vi "Current slew rate with scope.vi"() -> ()   [LabVIEW 2021]
uses:
  <instrlib>/niDCPower/nidcpower.llb/niDCPower Wait For Event - Event.ctl
  <instrlib>/niDCPower/nidcpower.llb/niDCPower Source Mode.ctl
  <instrlib>/niDCPower/nidcpower.llb/niDCPower Output Function.ctl
  <instrlib>/niDCPower/nidcpower.llb/niDCPower Aperture Time Units.ctl
  <instrlib>/niScope/Controls/niScope trigger slope.ctl
  <instrlib>/niScope/Utility/niScope Get Channel Name From String.vi
  <instrlib>/niScope/Configure/Trigger/niScope Configure Trigger Digital.vi
  <instrlib>/niDCPower/nidcpower.llb/niDCPower Configure Digital Edge Measure Trigger With Channels.vi
  <instrlib>/niScope/Acquire/Fetch/niScope Fetch WDT.vi
panel:
  in  "MeasGraphs":T1(tab)
  out "CurrentV/STime":waveform(dbl)(graph) caption="Load Transient"
  in  "SourceOutput Voltage v/s Time":string="SOURCE VOLTAGE vs TIME"
  out "ScopeAmplitudeV/STime":waveform(dbl)(graph) caption="Load Transient"
  in  "ScopeOutput Voltage v/s Time":string="SCOPE AMPLITUDE vs TIME"
  in  "error in":errorcluster caption="error in (no error)"
  out "error out":errorcluster
  in  "Source transient response":i32(ring)=1041 items=["Slow"=1041, "Normal"=1038, "Fast"=1039, "Custom"=1042]
  in  "MeasConfigurations":enum32{"Source Config", "Scope Config"}(tab)
  in  "TransientResponseTab":T2(tab)
  in  "Transient response":enum16{"Slow", "Normal", "Fast", "Custom"}(ring)=enum."Fast" caption="TRANSIENT RESPONSE"
  in  "Source current gain bandwidth":dbl=2000.0 caption="GAIN BANDWIDTH" format="%#_6pHz"
  in  "Source current compensation frequency":dbl=3530.0 caption="COMP. FREQUENCY" format="%#_6pHz"
  in  "Source current pole-zero ratio":dbl=2.0 caption="POLE-ZERO RATIO"
  in  "Source update rate":dbl=100000.0 caption="UPDATE RATE" format="%#_6pS/s"
  in  "Source sense":i32(ring)=1009 caption="SENSE" items=["Local"=1008, "Remote"=1009]
  in  "Source current C2 time":dbl=0.005 caption="TIME for C2" format="%#_6ps"
  in  "Source current C1 time":dbl=0.005 caption="TIME for C1" format="%#_6ps"
  in  "Source current slew rate":dbl=500.0 caption="CURRENT SLEW RATE" format="%#_6pA/s"
  in  "Source voltage limit range":dbl=20.0 caption="VOLTAGE LIMIT RANGE" format="%#_6pV"
  in  "Source current level range":dbl=3.0 caption="CURRENT LEVEL RANGE" format="%#_6pA"
  in  "Source current set point 2(C2)":dbl=3.0 caption="CURRENT SET POINT 2" format="%#_6pA"
  in  "Source current set point 1(C1)":dbl caption="CURRENT SET POINT 1" format="%#_6pA"
  in  "Source resource name":refnum<k15> caption="RESOURCE NAME"
  in  "Source SourceAdapt":string="Voltage SourceAdapt Parameters"
  in  "Source sample rate":dbl=1800000.0 caption="SAMPLE RATE" format="%#_6pS/s"
  in  "Scope enable/disable":bool caption="Scope Enable/Disable"
  in  "Scope vertical range":dbl=10.0 caption="VERTICAL RANGE"
  in  "Scope resourceName":refnum<k15> caption="RESOURCE NAME"
  in  "Scope probe attenuation":dbl=1.0 caption="PROBE ATTENUATION"
  in  "Scope sample rate":dbl=1800000.0 caption="SAMPLE RATE" format="%#_6pHz"
  in  "Scope output channel name":string="0" caption="INPUT CHANNEL NAME"
  in  "Scope vertical coupling":enum32{"AC", "DC"}(ring)=enum."DC" caption="VERTICAL COUPLING"
  # "CURRENT SLEW RATE"
  # "-"
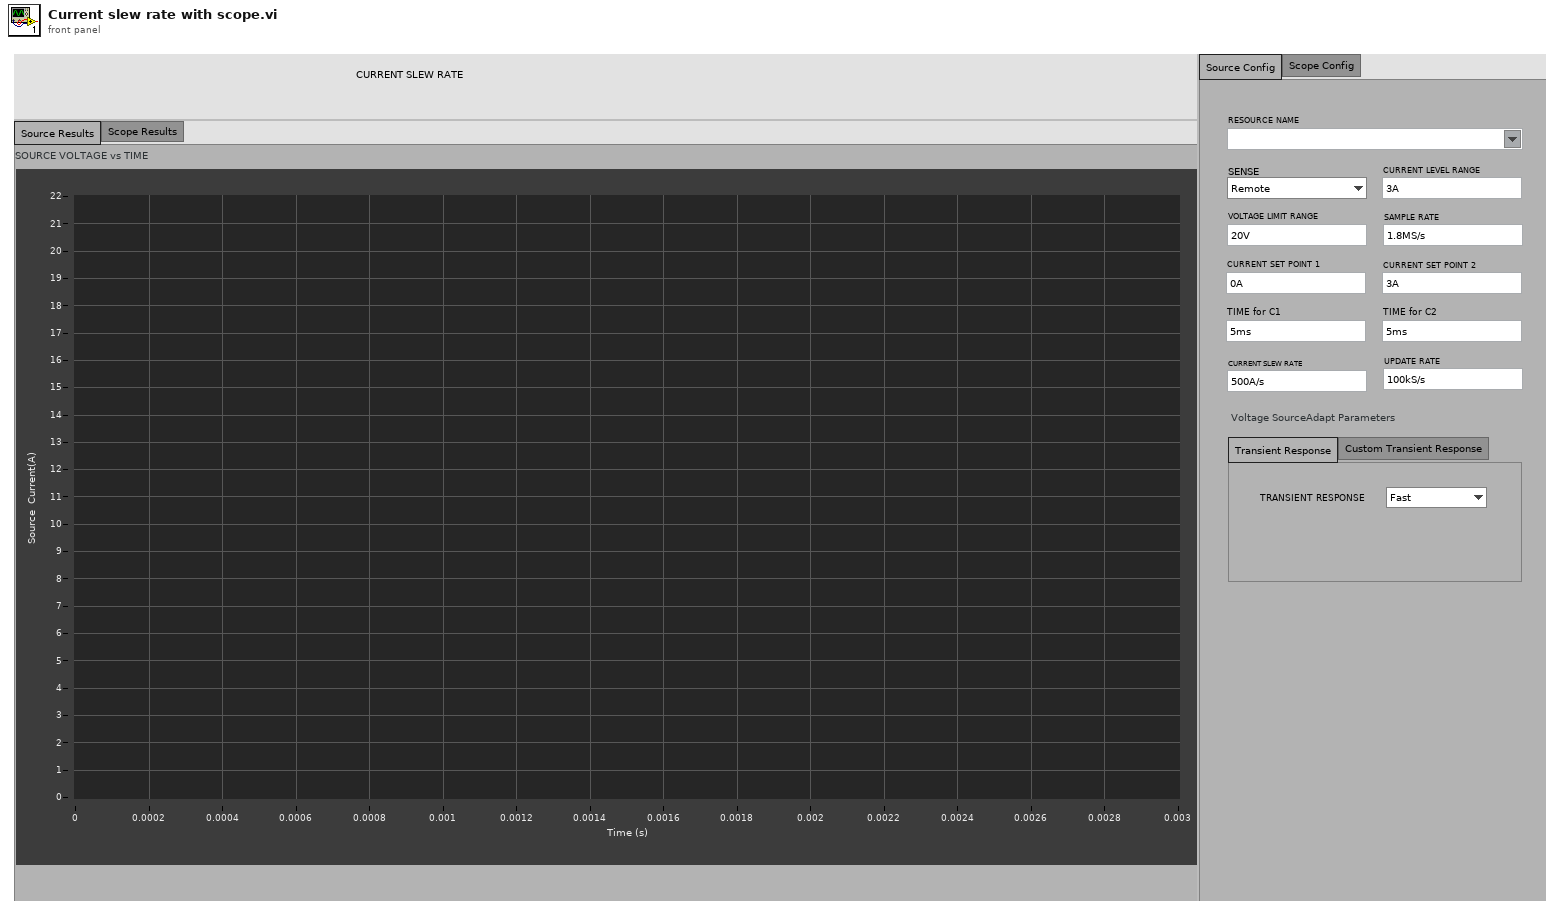
[diagram p1: front panel]
types:
  T1 = enum32{"Source Results", "Scope Results", "Hidden Controls"}
  T2 = enum32{"Transient Response", "Custom Transient Response"}
  T3 = typedef "niDCPower Aperture Time Units.ctl" = i32
  T4 = typedef "niDCPower Output Function.ctl" = i32
  T5 = typedef "niDCPower Wait For Event - Event.ctl" = i32
  T6 = typedef "niDCPower Source Mode.ctl" = i32
  T7 = typedef "niScope trigger slope.ctl" = i32
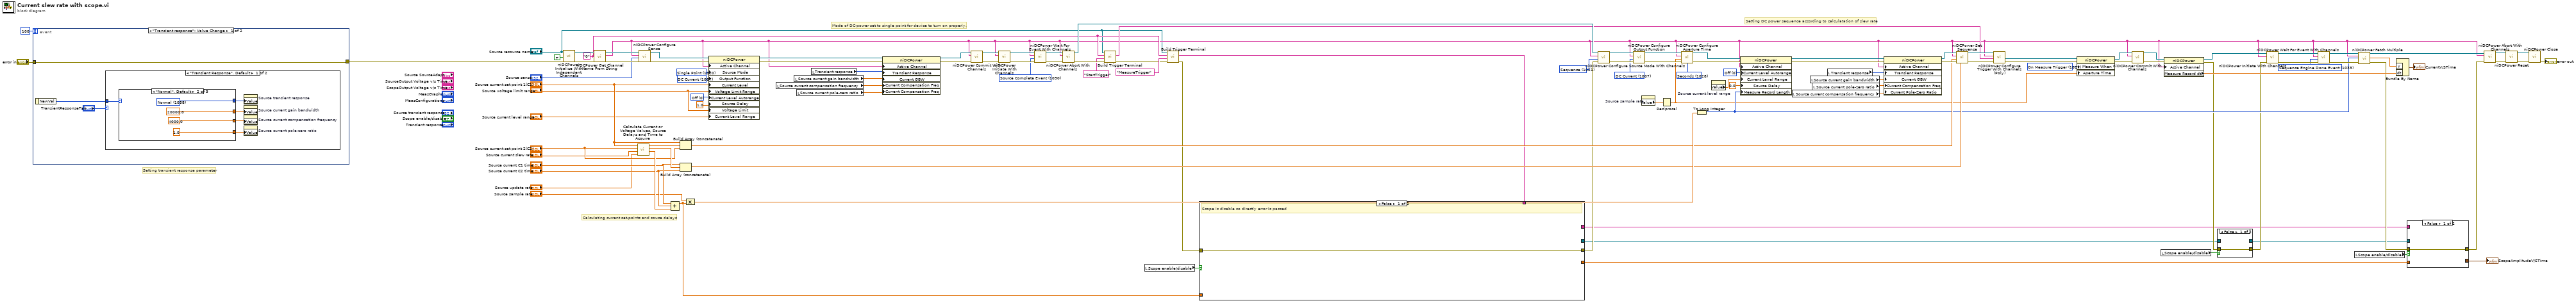
[diagram p0: block diagram]
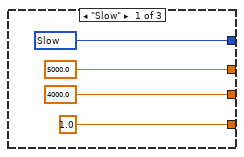
[diagram p2: hidden frame]
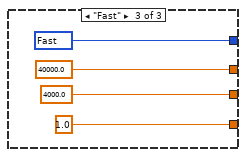
[diagram p3: hidden frame]
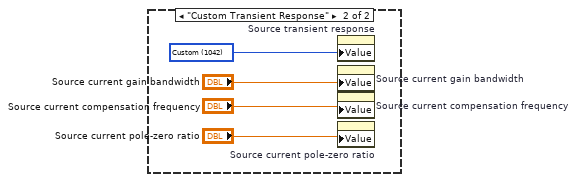
[diagram p4: hidden frame]
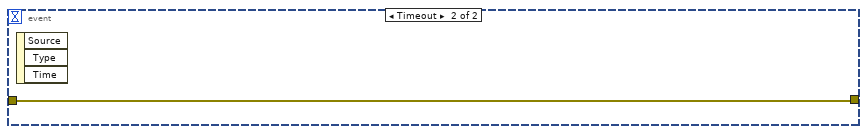
[diagram p5: hidden frame]
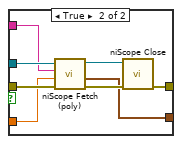
[diagram p6: hidden frame]
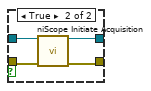
[diagram p7: hidden frame]
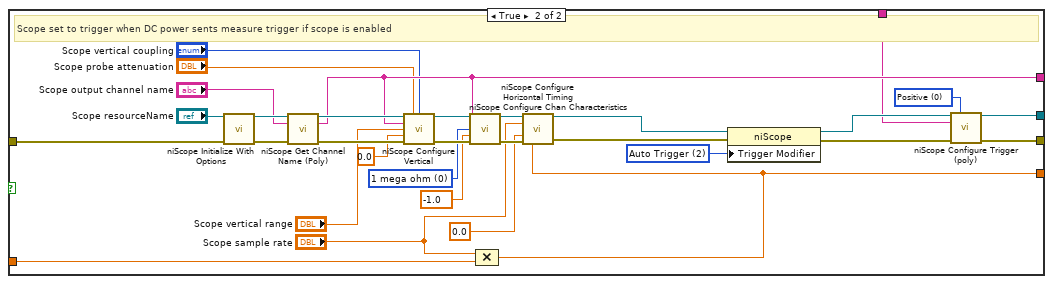
[diagram p8: hidden frame]
diagram:
  w73 = 1027 items=["Automatically after Source Complete"=1025, "On Demand"=1026, "On Measure Trigger"=1027] ("Measurement:Advanced:Measure When")
  w76 = 0 items=["Off", "On"] ("Source:DC Current:Current Level Autorange")
  w81 = T3 1028 items=["Seconds"=1028, "Powerline Cycles"=1029] ("aperture time units")
  w80 = T4 1007 items=["DC Voltage"=1006, "DC Current"=1007, "Pulse Voltage"=1049, "Pulse Current"=1050] ("output function")
  w82 = T5 1033 items=["Source Complete Event"=1030, "Measure Complete Event"=1031, "Sequence Iteration Complete Event"=1032, "Sequence Engine Done Event"=1033, "Pulse Complete Event"=1051, "Ready For Pulse Trigger Event"=1052] ("event")
  w83 = T6 1021 items=["Single Point"=1020, "Sequence"=1021] ("source mode")
  w44 = "0" ("index")
  w104 = 0 items=["Off", "On"] ("Source:DC Current:Current Level Autorange")
  w113 = T5 1030 items=["Source Complete Event"=1030, "Measure Complete Event"=1031, "Sequence Iteration Complete Event"=1032, "Sequence Engine Done Event"=1033, "Pulse Complete Event"=1051, "Ready For Pulse Trigger Event"=1052] ("event")
  w116 = 1007 items=["DC Voltage"=1006, "DC Current"=1007, "Pulse Voltage"=1049, "Pulse Current"=1050] ("Source:Output Function")
  w117 = 1020 items=["Single Point"=1020, "Sequence"=1021] ("Source:Source Mode")
  # "Calculating current set-points and souce delays"
  # "Setting DC power sequence according to calculatation of slew rate"
  # "Mode of DC-power set to single point for device to turn on properly."
  # "Setting transient response parameter"
  n1 = event shown="[0] \"Transient response\": Value Change" {
    selector: _ -> [_ _]
    dyn-events: _ -> [_ _]
    timeout: 100 -> [_ _]
    tunnel: [w120 w142] -> w1
    tunnel: "error in" -> [w120 w142]
    event "Transient response": Value Change {
      n2 = event-data() -> ("NewVal"=w119:enum16{"Slow", "Normal", "Fast", "Custom"})  [unwired: 1 in]
      n3 = case shown="\"Transient Response\", Default" "TransientResponseTab" {
        tunnel: w119 -> [w121 _]
        frame "Transient Response", Default {
          n4 = case shown="\"Normal\", Default" w121 {
            tunnel: [w129 w133 w137] -> w125
            tunnel: [5000.0 ("Source voltage gain bandwidth") 20000.0 ("Source voltage gain bandwidth") 40000.0 ("Source voltage gain bandwidth")] -> w124
            tunnel: [4000.0 ("Source voltage compensation frequency") 4000.0 ("Source voltage compensation frequency") 4000.0 ("Source voltage compensation frequency")] -> w122
            tunnel: [1.0 ("Source voltage pole-zero ratio") 1.0 ("Source voltage pole-zero ratio") 1.0 ("Source voltage pole-zero ratio")] -> w123
            frame "Slow" {
              w129 = 1041 items=["Slow"=1041, "Normal"=1038, "Fast"=1039, "Custom"=1042] ("Source transient response")
            }
            frame "Normal", Default {
              w133 = 1038 items=["Slow"=1041, "Normal"=1038, "Fast"=1039, "Custom"=1042] ("Source transient response")
            }
            frame "Fast" {
              w137 = 1039 items=["Slow"=1041, "Normal"=1038, "Fast"=1039, "Custom"=1042] ("Source transient response")
            }
          }
          n5 = property on="Source transient response" class="Ring (strict)"("Value"=w125) -> ()  [unwired: 2 in, 2 out]
          n6 = property on="Source current gain bandwidth" class="DigNum (strict)"("Value"=w124) -> ()  [unwired: 2 in, 2 out]
          n7 = property on="Source current compensation frequency" class="DigNum (strict)"("Value"=w122) -> ()  [unwired: 2 in, 2 out]
          n8 = property on="Source current pole-zero ratio" class="DigNum (strict)"("Value"=w123) -> ()  [unwired: 2 in, 2 out]
        }
        frame "Custom Transient Response" {
          w141 = 1042 items=["Slow"=1041, "Normal"=1038, "Fast"=1039, "Custom"=1042] ("Source transient response")
          n9 = property on="Source transient response" class="Ring (strict)"("Value"=w141) -> ()  [unwired: 2 in, 2 out]
          n10 = property on="Source current gain bandwidth" class="DigNum (strict)"("Value"="Source current gain bandwidth") -> ()  [unwired: 2 in, 2 out]
          n11 = property on="Source current compensation frequency" class="DigNum (strict)"("Value"="Source current compensation frequency") -> ()  [unwired: 2 in, 2 out]
          n12 = property on="Source current pole-zero ratio" class="DigNum (strict)"("Value"="Source current pole-zero ratio") -> ()  [unwired: 2 in, 2 out]
        }
      }
    }
    event Timeout {
      n13 = event-data() -> ()  [unwired: 1 in, 3 out]
    }
  }
  n14 = call <instrlib>:"niDCPower Initialize With Independent Channels.vi"("error in (no error)"=w1, "reset (false)"=TRUE, "resource name"="Source resource name") -> ("error out"=w98:errorcluster, "instrument handle out"=w101:refnum<k15>)  [unwired: 7 in]
  n15 = call <instrlib>:"niDCPower Get Channel Name From String.vi"("error in (no error)"=w98, "index"=w44, "instrument handle"=w101) -> ("error out"=w99:errorcluster, "name"=w37:string, "instrument handle out"=w100:refnum<k15>)  [unwired: 6 in]
  n16 = call "Calculate Current or Voltage Values, Source Delays and Time to Acquire.vi"("Update Rate (S/sec)"="Source update rate", "Current/voltage slew rate (AorV/sec)"="Source current slew rate", "Current/voltage end point (A/V)"="Source current set point 2(C2)", "Current/voltage start point  (A/V)"="Source current set point 1(C1)") -> ("Time to acquire (sec)"=w36:dbl, "Source delays (sec)"=w35:dbl[], "Current/voltage values"=w34:dbl[])  [unwired: 5 in]
  n17 = call <instrlib>:"niDCPower Configure Sense.vi"("error in (no error)"=w99, "sense"="Source sense", "channel name"=w37, "instrument handle"=w100) -> ("error out"=w109:errorcluster, "instrument handle out"=w110:refnum<k15>)  [unwired: 6 in]
  n18 = Compound Arithmetic op=ADD("Source current C1 time", "Source current C2 time", w36) -> (w47:dbl)
  n19 = Build Array (concatenate)("Source current set point 1(C1)", w34, "Source current set point 2(C2)") -> (w66:dbl[])
  n20 = Build Array (concatenate)("Source current C1 time", w35, "Source current C2 time") -> (w67:dbl[])
  n21 = Compound Arithmetic op=MULTIPLY("Source sample rate", w47) -> (w90:dbl)
  n22 = property class="niDCPower"(reference=w110, error in=w109, "Active Channel"=w37, "Source Mode"=w117, "Output Function"=w116, "Current Level"="Source current set point 1(C1)", "Voltage Limit Range"="Source voltage limit range", "Current Level Autorange"=w104, "Source Delay"=1.0 ("Source:Advanced:Source Delay"), "Voltage Limit"="Source voltage limit range", "Current Level Range"="Source current level range") -> (reference out=w106:refnum<k15>, error out=w105:errorcluster)
  n23 = local read "Source current compensation frequency"() -> (w12:dbl)
  n24 = local read "Source current gain bandwidth"() -> (w13:dbl)
  n25 = local read "Source current pole-zero ratio"() -> (w11:dbl)
  n26 = local read "Transient response"() -> (w10:enum16{"Slow", "Normal", "Fast", "Custom"})
  n27 = property class="niDCPower"(reference=w106, error in=w105, "Active Channel"=w37, "Transient Response"=w10, "Current GBW"=w13, "Current Compensation Freq"=w12, "Current Compensation Freq"=w11) -> (reference out=w103:refnum<k15>, error out=w102:errorcluster)
  n28 = call <instrlib>:"niDCPower Commit With Channels.vi"("error in (no error)"=w102, "channel name"=w37, "instrument handle"=w103) -> ("error out"=w107:errorcluster, "instrument handle out"=w108:refnum<k15>)  [unwired: 7 in]
  n29 = call <instrlib>:"niDCPower Initiate With Channels.vi"("error in (no error)"=w107, "channel name"=w37, "instrument handle"=w108) -> ("error out"=w115:errorcluster, "instrument handle out"=w114:refnum<k15>)  [unwired: 7 in]
  n30 = call <instrlib>:"niDCPower Wait For Event With Channels.vi"("error in (no error)"=w115, "event"=w113, "channel name"=w37, "instrument handle"=w114) -> ("error out"=w112:errorcluster, "instrument handle out"=w111:refnum<k15>)  [unwired: 6 in]
  n31 = call <instrlib>:"niDCPower Abort With Channels.vi"("error in (no error)"=w112, "channel name"=w37, "instrument handle"=w111) -> ("error out"=w58:errorcluster, "instrument handle out"=w68:refnum<k15>)  [unwired: 7 in]
  n32 = call "Build Trigger Terminal.vi"("error in (no error)"=w58, "Trigger/Event Name"="StartTrigger" ("Trigger Type"), "Channel Name"=w44, "Resource Name"="Source resource name") -> ("error out"=w30:errorcluster, "Terminal Name"=w57:string)  [unwired: 6 in]
  n33 = local read "Scope enable/disable"() -> (w15:bool)
  n34 = call "Build Trigger Terminal.vi"("error in (no error)"=w30, "Trigger/Event Name"="MeasureTrigger", "Channel Name"=w44, "Resource Name"="Source resource name") -> ("error out"=w45:errorcluster, "Terminal Name"=w33:string)  [unwired: 6 in]
  n35 = case shown="False" w15 {
    tunnel: [w143 w156] -> w55
    tunnel: [_ w155] -> w50
    tunnel: [_ w154] -> w48
    tunnel: w47 -> [_ w153]
    tunnel: [_ w152] -> w46
    tunnel: w45 -> [w143 w151]
    tunnel: w33 -> [_ w150]
    frame False {
      # "Scope is disable so directly error is passed"
    }
    frame True {
      w163 = 2 items=["None"=1, "Auto Trigger"=2] ("Trigger Modifier")
      w159 = u32 0 items=["1 mega ohm"=0, "50 ohms"=2] ("Input Impedance")
      w160 = T7 0 items=["Positive", "Negative"] ("trigger slope")
      # "Scope set to trigger when DC power sents measure trigger if scope is enabled"
      n36 = call <instrlib>:"niScope Initialize With Options.vi"("resource name"="Scope resourceName", "error in"=w151) -> ("instrument handle"=w174:refnum<k15>, "error out"=w173:errorcluster)  [unwired: 12 in]
      n37 = call-poly <instrlib>:"niScope Get Channel Name (Poly).vi"("instrument handle"=w174, "index"="Scope output channel name", "error in"=w173) -> ("instrument handle out"=w162:refnum<k15>, "channel name"=w154:string, "error out"=w161:errorcluster)  [unwired: 10 in]
      n38 = call <instrlib>:"niScope Configure Vertical.vi"("instrument handle"=w162, "probe attenuation"="Scope probe attenuation", "vertical coupling"="Scope vertical coupling", "channels"=w154, "vertical range"="Scope vertical range", "vertical offset"=0.0, "error in"=w161) -> ("instrument handle out"=w172:refnum<k15>, "error out"=w171:errorcluster)  [unwired: 7 in]
      n39 = call <instrlib>:"niScope Configure Chan Characteristics.vi"("instrument handle"=w172, "channels"=w154, "input impedance"=w159, "maximum input frequency"=-1.0 ("Maximum Input Frequency"), "error in"=w171) -> ("instrument handle out"=w169:refnum<k15>, "error out"=w170:errorcluster)  [unwired: 9 in]
      n40 = Compound Arithmetic op=MULTIPLY("Scope sample rate", w153) -> (w152:dbl)
      n41 = call <instrlib>:"niScope Configure Horizontal Timing.vi"("instrument handle"=w169, "min sample rate"="Scope sample rate", "reference position"=0.0 ("Reference Position"), "error in"=w170, "min record length"=w152) -> ("instrument handle out"=w166:refnum<k15>, "error out"=w165:errorcluster)  [unwired: 9 in]
      n42 = property on="Property Node" class="niScope"(reference=w166, error in=w165, "Trigger Modifier"=w163) -> (reference out=w157:refnum<k15>, error out=w164:errorcluster)
      n43 = call-poly <instrlib>:"niScope Configure Trigger (poly).vi"("instrument handle"=w157, "trigger slope"=w160, "trigger source"=w150, "error in"=w164) -> ("instrument handle out"=w155:refnum<k15>, "error out"=w156:errorcluster)  [unwired: 10 in]
    }
  }
  n44 = call <instrlib>:"niDCPower Configure Source Mode With Channels.vi"("error in (no error)"=w55, "source mode"=w83, "channel name"=w37, "instrument handle"=w68) -> ("error out"=w86:errorcluster, "instrument handle out"=w85:refnum<k15>)  [unwired: 6 in]
  n45 = call <instrlib>:"niDCPower Configure Output Function.vi"("error in (no error)"=w86, "output function"=w80, "channel name"=w37, "instrument handle"=w85) -> ("error out"=w88:errorcluster, "instrument handle out"=w87:refnum<k15>)  [unwired: 6 in]
  n46 = property on="Source sample rate" class="DigNum (strict)"() -> ("Value"=w2:dbl)  [unwired: 2 in, 2 out]
  n47 = Reciprocal(x=w2) -> (1/x=w32:dbl)
  n48 = call <instrlib>:"niDCPower Configure Aperture Time.vi"("aperture time units"=w81, "error in (no error)"=w88, "aperture time"=w32, "channel name"=w37, "instrument handle"=w87) -> ("error out"=w78:errorcluster, "instrument handle out"=w77:refnum<k15>)  [unwired: 5 in]
  n49 = To Long Integer(number=w90) -> (32bit integer=w63:i32)
  n50 = property on="Source current level range" class="DigNum (strict)"() -> ("Value"=w3:dbl)  [unwired: 2 in, 2 out]
  n51 = property class="niDCPower"(reference=w77, error in=w78, "Active Channel"=w37, "Current Level Autorange"=w76, "Current Level Range"=w3, "Source Delay"=0.0 ("Source:Advanced:Source Delay"), "Measure Record Length"=w63) -> (reference out=w94:refnum<k15>, error out=w95:errorcluster)
  n52 = local read "Source current compensation frequency"() -> (w7:dbl)
  n53 = local read "Source current gain bandwidth"() -> (w9:dbl)
  n54 = local read "Source current pole-zero ratio"() -> (w8:dbl)
  n55 = local read "Transient response"() -> (w14:enum16{"Slow", "Normal", "Fast", "Custom"})
  n56 = property class="niDCPower"(reference=w94, error in=w95, "Active Channel"=w37, "Transient Response"=w14, "Current GBW"=w9, "Current Compensation Freq"=w8, "Current Pole-Zero Ratio"=w7) -> (reference out=w96:refnum<k15>, error out=w97:errorcluster)
  n57 = call <instrlib>:"niDCPower Set Sequence.vi"("source delays"=w67, "error in (no error)"=w97, "values"=w66, "channel name"=w37, "instrument handle"=w96) -> ("error out"=w74:errorcluster, "instrument handle out"=w75:refnum<k15>)  [unwired: 5 in]
  n58 = call-poly <instrlib>:"niDCPower Configure Trigger With Channels (Poly).vi"("error in (no error)"=w74, "input terminal"=w57, "channel name"=w37, "instrument handle"=w75) -> ("error out"=w70:errorcluster, "instrument handle out"=w72:refnum<k15>)  [unwired: 6 in]
  n59 = property class="niDCPower"(reference=w72, error in=w70, "Measure When"=w73, "Aperture Time"=w32) -> (reference out=w71:refnum<k15>, error out=w69:errorcluster)
  n60 = call <instrlib>:"niDCPower Commit With Channels.vi"("error in (no error)"=w69, "channel name"=w37, "instrument handle"=w71) -> ("error out"=w93:errorcluster, "instrument handle out"=w89:refnum<k15>)  [unwired: 7 in]
  n61 = local read "Scope enable/disable"() -> (w17:bool)
  n62 = property class="niDCPower"(reference=w89, error in=w93, "Active Channel"=w37) -> (reference out=w84:refnum<k15>, error out=w54:errorcluster, "Measure Record dt"=w61:dbl)
  n63 = case shown="False" w17 {
    tunnel: w54 -> [w175 w179]
    tunnel: [w175 w178] -> w53
    tunnel: w50 -> [_ w177]
    tunnel: [_ w176] -> w49
    frame False {
    }
    frame True {
      n64 = call <instrlib>:"niScope Initiate Acquisition.vi"("instrument handle"=w177, "error in"=w179) -> ("instrument handle out"=w176:refnum<k15>, "error out"=w178:errorcluster)  [unwired: 12 in]
    }
  }
  n65 = call <instrlib>:"niDCPower Initiate With Channels.vi"("error in (no error)"=w53, "channel name"=w37, "instrument handle"=w84) -> ("error out"=w92:errorcluster, "instrument handle out"=w91:refnum<k15>)  [unwired: 7 in]
  n66 = call <instrlib>:"niDCPower Wait For Event With Channels.vi"("error in (no error)"=w92, "event"=w82, "channel name"=w37, "instrument handle"=w91) -> ("error out"=w65:errorcluster, "instrument handle out"=w64:refnum<k15>)  [unwired: 6 in]
  n67 = local read "Scope enable/disable"() -> (w16:bool)
  n68 = call <instrlib>:"niDCPower Fetch Multiple.vi"("instrument handle"=w64, "channel name"=w37, "count (1)"=w63, "error in (no error)"=w65) -> ("instrument handle out"=w62:refnum<k15>, "current measurements"=w60:dbl[], "error out"=w52:errorcluster)  [unwired: 6 in, 3 out]
  n69 = Bundle By Name("Y"=w60, "dt"=w61) -> (→"CurrentV/STime":waveform(dbl))  [unwired: 1 in]
  n70 = case shown="False" w16 {
    tunnel: w52 -> [w180 w188]
    tunnel: [w180 w187] -> w51
    tunnel: w49 -> [_ w185]
    tunnel: w48 -> [_ w184]
    tunnel: w46 -> [_ w182]
    tunnel: [_ w181] -> w18
    frame False {
    }
    frame True {
      n71 = call-poly <instrlib>:"niScope Fetch (poly).vi"("error in"=w188, "numSamples"=w182, "channels"=w184, "instrument handle"=w185) -> ("error out"=w186:errorcluster, "wfm"=w181:waveform(dbl), "instrument handle out"=w183:refnum<k15>)  [unwired: 4 in, 1 out]
      n72 = call <instrlib>:"niScope Close.vi"("instrument handle"=w183, "error in"=w186) -> ("error out"=w187:errorcluster)  [unwired: 13 in]
    }
  }
  "ScopeAmplitudeV/STime" <- w18
  n73 = call <instrlib>:"niDCPower Abort With Channels.vi"("error in (no error)"=w51, "channel name"=w37, "instrument handle"=w62) -> ("error out"=w42:errorcluster, "instrument handle out"=w40:refnum<k15>)  [unwired: 7 in]
  n74 = call <instrlib>:"niDCPower Reset.vi"("error in (no error)"=w42, "instrument handle"=w40) -> ("error out"=w41:errorcluster, "instrument handle out"=w39:refnum<k15>)  [unwired: 8 in]
  n75 = call <instrlib>:"niDCPower Close.vi"("error in (no error)"=w41, "instrument handle"=w39) -> ("error out"=→"error out":errorcluster)  [unwired: 9 out]
